vi "SendTelnetCmd.vi"(6 "Target IP":string="192.168.1.1", 8 "error in":errorcluster, 9 "DelayAfterWrite":dbl=1000.0, 10 "Initial delay":dbl=25000.0, 11 "WriteData":string="\r") -> (0 "error out":errorcluster, 3 "Response":string=" ")   [LabVIEW 2013]
doc: "This VI implements a client for the named service created by Named Service TCP Server.vi.\nThe client connects to the service using the name of the service and the address of the server. It receives the response from the server, displays it and closes the connection.\n\n<b>Note:</b> This VI is built to work with the Named Service TCP Server.vi in TCP.llb."
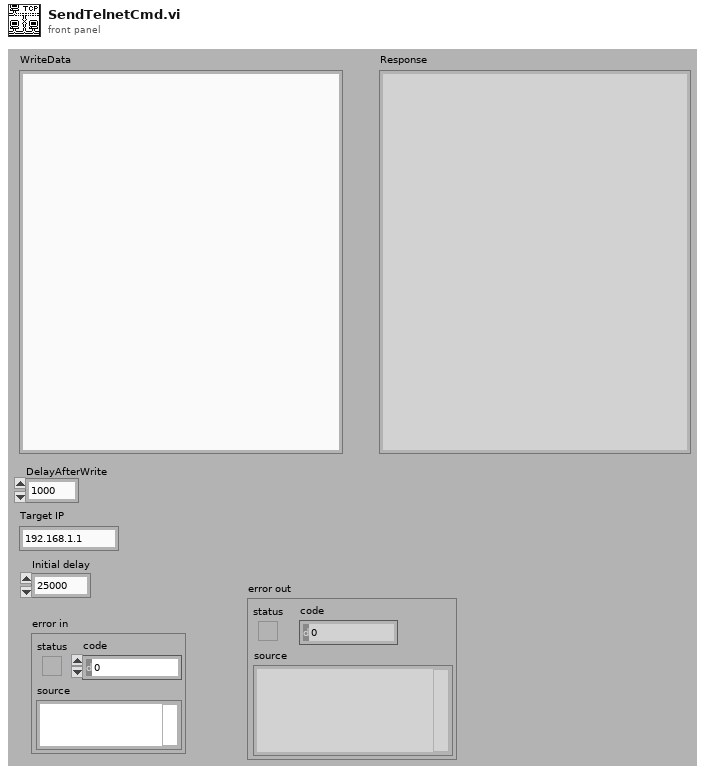
[diagram p1: front panel]
types:
  T1 = enum16{"Standard", "Buffered", "CRLF", "Immediate"}
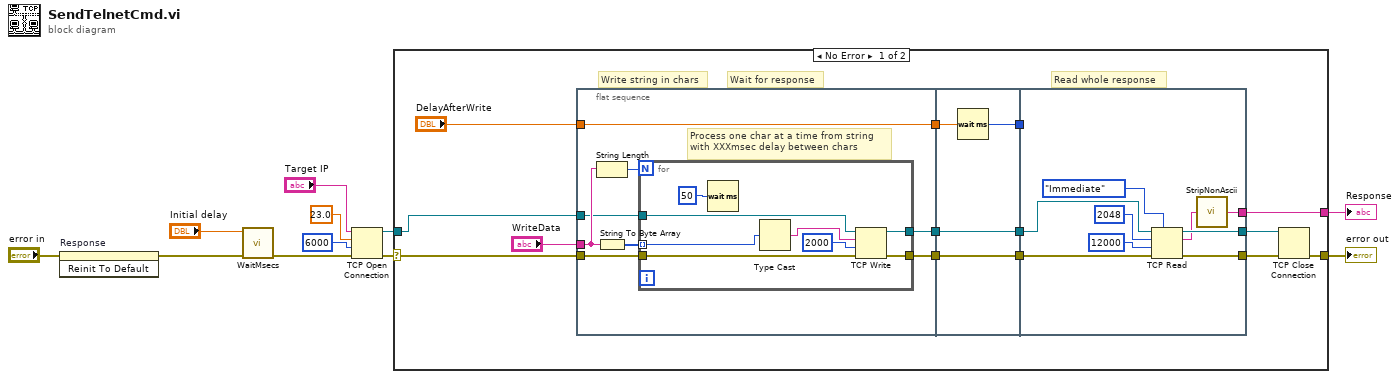
[diagram p0: block diagram]
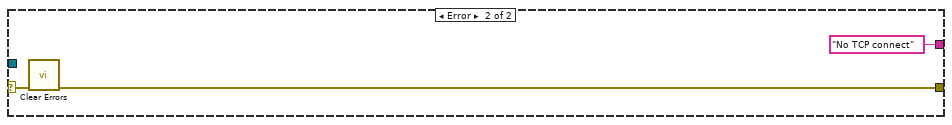
[diagram p2: hidden frame]
diagram:
  n1 = invoke on="Response" class="Str" method="Reinit To Default"(error in="error in") -> (error out=w7:errorcluster)  [unwired: 2 in, 2 out]
  n2 = call "WaitMsecs.vi"("error in (no error)"=w7, "Wait Msecs"="Initial delay") -> ("error out"=w4:errorcluster)  [unwired: 9 in]
  n3 = TCP Open Connection(address="Target IP", remote port or service name=23.0 ("TCP Port Number"), timeout ms (60000)=6000, error in (no error)=w4) -> (connection ID=w6:refnum<k5>, error out=w2:errorcluster)  [unwired: 1 in]
  n4 = case shown="No Error" w2 {
    selector: w2 -> [w13 w56]
    tunnel: [w17 w55] -> w10
    tunnel: w6 -> [w12 _]
    tunnel: [w14 "No TCP connect" ("Outgoing String")] -> w1
    frame No Error {
      # "Read whole response"
      # "Wait for response"
      # "Write string in chars"
      n5 = flat-sequence {
        tunnel: "WriteData" -> [w31]
        tunnel: [w26] -> w25
        tunnel: w12 -> [w30]
        tunnel: w13 -> [w29]
        tunnel: [w28] -> w24
        tunnel: [w27] -> w23
        tunnel: "DelayAfterWrite" -> [w26]
        tunnel: w25 -> [w45]
        tunnel: [w44] -> w22
        tunnel: w24 -> [w43]
        tunnel: [w43] -> w21
        tunnel: w23 -> [w42]
        tunnel: [w42] -> w20
        tunnel: w22 -> [_]
        tunnel: [w52] -> w19
        tunnel: w21 -> [w51]
        tunnel: w20 -> [w50]
        tunnel: [w49] -> w18
        tunnel: [w47] -> w14
        frame #0 {
          # "Process one char at a time from string\nwith XXXmsec delay between chars"
          n6 = String Length(string=w31) -> (length=w33:i32)
          n7 = String To Byte Array(string=w31) -> (unsigned byte array=w32:u8[])
          n8 = for {
            N: w33 -> [_]
            tunnel: w32 -> [w41] mode=indexing
            tunnel: w30 -> [w40]
            tunnel: w29 -> [w38]
            tunnel: [w37] -> w27
            tunnel: [w36] -> w28
            n9 = Wait (ms)(milliseconds to wait=u32 50) -> ()  [unwired: 1 out]
            n10 = Type Cast(x=w41) -> (*(type *) &x=w39:string)  [unwired: 1 in]
            n11 = TCP Write(connection ID=w40, data in=w39, error in (no error)=w38, 9:2000 ("timeout ms (25000)")) -> (connection ID out=w36:refnum<k5>, error out=w37:errorcluster)  [unwired: 1 out]
          }
        }
        frame #1 {
          n12 = Wait (ms)(milliseconds to wait=w45) -> (millisecond timer value=w44:u32)
        }
        frame #2 {
          n13 = TCP Read(connection ID=w51, bytes to read=2048, error in (no error)=w50, 7:T1."Immediate" ("mode (standard)"), 9:12000 ("timeout ms (25000)")) -> (connection ID out=w52:refnum<k5>, data out=w48:string, error out=w49:errorcluster)
          n14 = call "StripNonAscii.vi"("Incoming String"=w48) -> ("Outgoing String"=w47:string)
        }
      }
      n15 = TCP Close Connection(connection ID=w19, error in (no error)=w18) -> (error out=w17:errorcluster)  [unwired: 1 in, 1 out]
    }
    frame Error {
      n16 = call <vilib>:"Clear Errors.vi"("error in (no error)"=w56) -> ("error out"=w55:errorcluster)  [unwired: 6 in]
    }
  }
  "error out" <- w10
  "Response" <- w1
